vi "ServoControl_myrio_v3_measure.vi"() -> ()   [LabVIEW 2019]
uses:
  <vilib>/Platform/TimedLoop/XDataNode/timing_clust.ctl
  <vilib>/Platform/TimedLoop/XDataNode/nitl_modes.ctl
  <vilib>/Platform/TimedLoop/XDataNode/wakeup.ctl
  <vilib>/Instr/_visa.llb/VISA Configure Serial Port (Instr).vi
  <vilib>/Utility/file.llb/Write Delimited Spreadsheet (DBL).vi
  <vilib>/platform/TimedLoop/XDataNode/XDataNode.xnode
  <vilib>/Platform/TimedLoop/XDataNode/XDNodeRunTimeDep.lvlib
panel:
  in  "Period":dbl
  out "Position Chart":cluster{dbl, dbl}(graph)
  out "Position Graph":cluster{dbl[], dbl[]}[](graph)
  in  "plot freq.":i32=5
  in  "const(f)/sine(t)":bool
  out "iteration":i32
  out "time":dbl
  out "sine position":dbl
  out "read from visa":string
  out "write to visa":string
  in  "const posotion":dbl=180.0
  in  "format (%.3f)":string="%.3f"
  in  "file path (dialog if empty)":path
  in  "Period":i64=5
  in  "stop":bool
  in  "VISA resource name":refnum<visa-resource-name>="ASRL2::INSTR"
  in  "baud rate (9600)":u32=500000
  out "error out":errorcluster
  # "visa setting"
  # "measure time"
  # "status setting"
  # "File save"
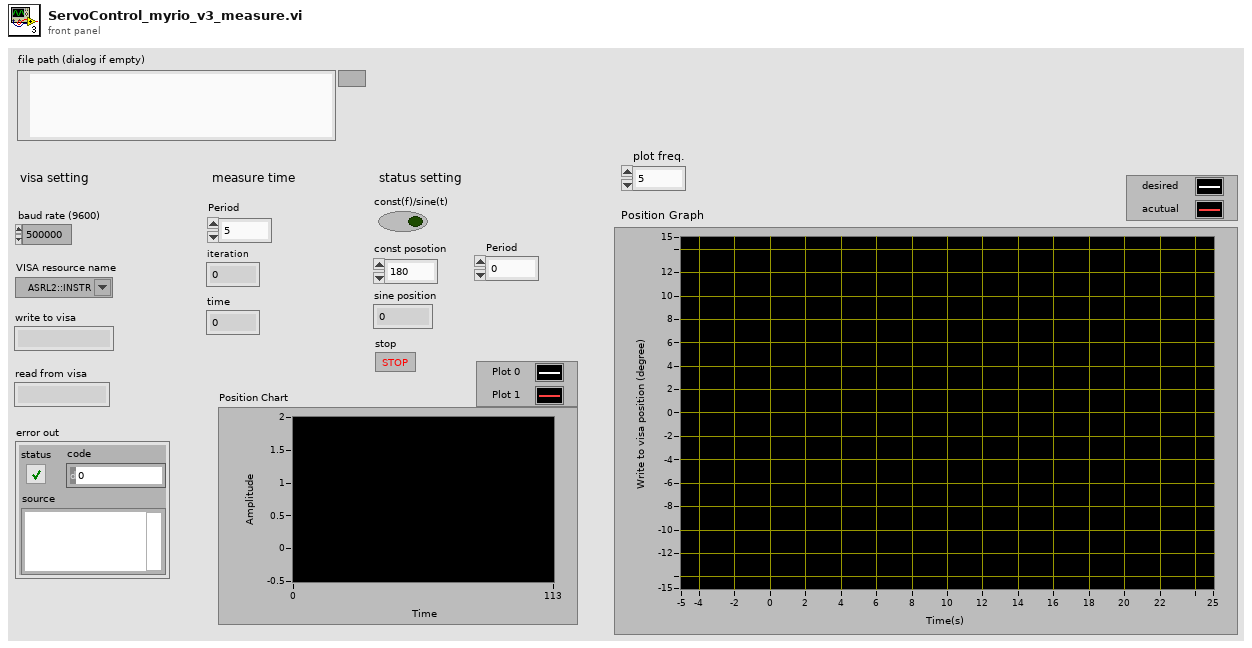
[diagram p1: front panel]
types:
  T1 = typedef "XDNodeRunTimeDep.lvlib/timing_clust.ctl" = cluster{"Expected End [f-1]":u64, "Actual End [f-1]":u64, "Finished Late? [f-1]":bool, "Expected End [i-1]":u64, "Actual End [i-1]":u64, "Finished Late? [i-1]":bool, "Expected Start [i]":u64, "Actual Start [i]":u64, "Expected Start [f]":u64, "Actual Start [f]":u64, "Source Name":string, "Structure Name":string, "Period":i64, "Deadline":i64, "Offset":i64, "Start":i64, "Priority":i32, "Timeout":i32, "Mode":T2, "Wakeup Reason":T3, "Error":errorcluster, "Source Type":string, "Secondary Source Type":string, "Global End Time":u64, "Global Start Time":u64, "Frame Duration":u64, "Iteration Duration":u64, "Assigned CPU":i32, "I/O Scan Engine Mode":u32}
  T2 = typedef "XDNodeRunTimeDep.lvlib/nitl_modes.ctl" = enum32{"No Change", "Process missed periods, maintain original phase", "Discard missed periods, maintain original phase", "Process missed periods, ignore original phase", "Discard missed periods, ignore original phase"}
  T3 = typedef "XDNodeRunTimeDep.lvlib/wakeup.ctl" = enum32{"Normal", "Aborted", "Asynchronous wakeup", "Timing source error", "Timed loop error", "Timeout"}
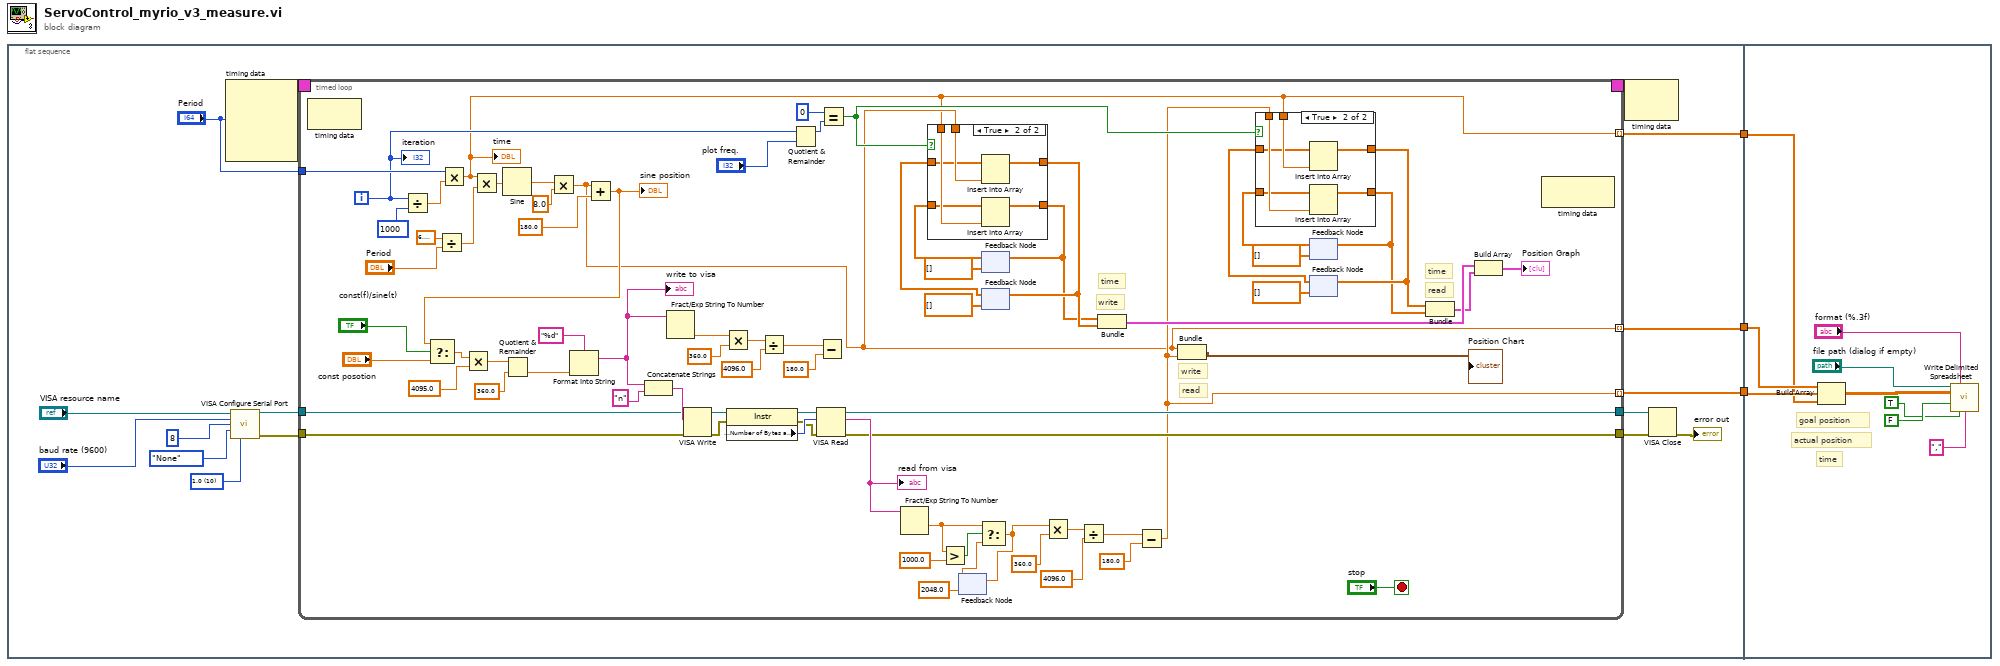
[diagram p0: block diagram]
diagram:
  n1 = flat-sequence {
    tunnel: [w7] -> w3
    tunnel: [w6] -> w2
    tunnel: [w5] -> w1
    tunnel: w3 -> [w118]
    tunnel: w2 -> [w117]
    tunnel: w1 -> [w116]
    frame #0 {
      w14 = u16 10 items=["1.0"=10, "1.5"=15, "2.0"=20] ("stop bits (10: 1 bit)")
      n2 = node-c288("Period") -> (w19:T1)  [unwired: 3 in]
      n3 = call-poly "VISA Configure Serial Port"("VISA resource name"="VISA resource name", "baud rate (9600)"="baud rate (9600)", "data bits (8)"=u16 8, "parity (0:none)"=enum16{"None", "Odd", "Even", "Mark", "Space"}."None", "stop bits (10: 1 bit)"=w14) -> ("VISA resource name out"=w13:refnum<visa-resource-name>, "error out"=w12:errorcluster)  [unwired: 9 in]
      n4 = timed-loop {
        timing: w19 -> [_]
        timing-out: [_] -> w18
        tunnel: "Period" -> [w35]
        tunnel: w12 -> [w36]
        tunnel: [w33] -> w11
        tunnel: w13 -> [w37]
        tunnel: [w32] -> w4
        tunnel: [w30] -> w7 mode=indexing
        tunnel: [w31] -> w6 mode=indexing
        tunnel: [w29] -> w5 mode=indexing
        i -> [w34]
        stop <- "stop" stop-if-true
        # "time"
        # "read"
        # "time"
        # "write"
        # "read"
        # "write"
        n5 = node-c288() -> ()  [unwired: 1 in, 1 out]
        n6 = Divide(x=w34, y=i64 1000) -> (x/y=w70:dbl)
        n7 = Divide(x=6.283185307179586, y="Period") -> (x/y=w20:dbl)
        n8 = Multiply(x=w35, y=w70) -> (x*y=w29:dbl)
        "time" <- w29
        n9 = Multiply(x=w29, y=w20) -> (x*y=w73:dbl)
        n10 = Sine(x=w73) -> (sin(x)=w56:dbl)
        n11 = Multiply(x=w56, y=8.0) -> (x*y=w30:dbl)
        n12 = Add(x=w30, y=180.0) -> (x+y=w68:dbl)
        "sine position" <- w68
        n13 = Select(t=w68, s="const(f)/sine(t)", f="const posotion") -> (s? t:f=w66:dbl)
        n14 = Multiply(x=w66, y=4095.0) -> (x*y=w90:dbl)
        n15 = Quotient & Remainder(x=w90, y=360.0) -> (floor(x/y)=w88:dbl)  [unwired: 1 out]
        n16 = Format Into String(format string="%d", w88) -> (resulting string=w80:string)  [unwired: 2 in, 1 out]
        "write to visa" <- w80
        n17 = Concatenate Strings(w80, "n" ("string")) -> (w92:string)
        n18 = Fract/Exp String To Number(string=w80) -> (number=w79:dbl)  [unwired: 3 in, 1 out]
        n19 = VISA Write(VISA resource name=w37, write buffer=w92, error in (no error)=w36) -> (VISA resource name out=w54:refnum<visa-resource-name>, error out=w53:errorcluster)  [unwired: 1 out]
        n20 = Multiply(x=w79, y=360.0 ("x")) -> (x*y=w77:dbl)
        n21 = property class="Instr"(reference=w54, error in=w53) -> (reference out=w51:refnum<visa-resource-name>, error out=w50:errorcluster, "Serial Settings:Number of Bytes at Serial Port"=w52:u32)
        n22 = Divide(x=w77, y=4096.0) -> (x/y=w83:dbl)
        n23 = Quotient & Remainder(x=w34, y="plot freq.") -> (x-y*floor(x/y)=w61:i32)  [unwired: 1 out]
        n24 = VISA Read(VISA resource name=w51, byte count=w52, error in (no error)=w50) -> (VISA resource name out=w32:refnum<visa-resource-name>, read buffer=w81:string, error out=w33:errorcluster)  [unwired: 1 out]
        "read from visa" <- w81
        n25 = Subtract(x=w83, y=180.0) -> ()  [unwired: 1 out]
        n26 = Equal?(x=0, y=w61) -> (x = y?=w40:bool)
        n27 = Fract/Exp String To Number(string=w81) -> (number=w49:dbl)  [unwired: 3 in, 1 out]
        n28 = Greater?(x=w49, y=1000.0) -> (0:w48:bool)
        n29 = feedback #1(2048.0) -> (w24:dbl)
        n30 = Select(t=w49, s=w48, f=w24) -> (s? t:f=w25:dbl)
        n31 = feedback-in #1(w25) -> ()
        n32 = feedback #2(dbl[] []) -> (w65:dbl[])
        n33 = feedback #3(dbl[] []) -> (w62:dbl[])
        n34 = case shown="True" w40 {
          tunnel: w30 -> [_ w109]
          tunnel: w29 -> [_ w108]
          tunnel: [w103 w107] -> w57
          tunnel: w65 -> [w103 w106]
          tunnel: [w102 w105] -> w58
          tunnel: w62 -> [w102 w104]
          frame False {
          }
          frame True {
            n35 = Insert Into Array(array=w104, new element=w109) -> (w105:dbl[])  [unwired: 1 in]
            n36 = Insert Into Array(array=w106, new element=w108) -> (w107:dbl[])  [unwired: 1 in]
          }
        }
        n37 = feedback-in #2(w57) -> ()
        n38 = feedback-in #3(w58) -> ()
        n39 = Multiply(x=w25, y=360.0 ("x")) -> (x*y=w74:dbl)
        n40 = Divide(x=w74, y=4096.0) -> (x/y=w76:dbl)
        n41 = Bundle(w57, w58) -> (w43:cluster{dbl[], dbl[]})  [unwired: 1 in]
        n42 = Subtract(x=w76, y=180.0) -> (x-y=w31:dbl)
        n43 = Bundle(w30, w31) -> (→"Position Chart":cluster{dbl, dbl})  [unwired: 1 in]
        n44 = feedback #4(dbl[] []) -> (w47:dbl[])
        n45 = feedback #5(dbl[] []) -> (w44:dbl[])
        n46 = case shown="True" w40 {
          tunnel: w29 -> [_ w101]
          tunnel: w31 -> [_ w100]
          tunnel: [w95 w99] -> w38
          tunnel: w47 -> [w95 w98]
          tunnel: [w94 w97] -> w39
          tunnel: w44 -> [w94 w96]
          frame False {
          }
          frame True {
            n47 = Insert Into Array(array=w96, new element=w101) -> (w97:dbl[])  [unwired: 1 in]
            n48 = Insert Into Array(array=w98, new element=w100) -> (w99:dbl[])  [unwired: 1 in]
          }
        }
        n49 = feedback-in #4(w38) -> ()
        n50 = feedback-in #5(w39) -> ()
        n51 = Bundle(w39, w38) -> (w42:cluster{dbl[], dbl[]})  [unwired: 1 in]
        n52 = Build Array(w43, w42) -> (→"Position Graph":cluster{dbl[], dbl[]}[])
        n53 = node-c288() -> ()  [unwired: 1 in, 1 out]
        "iteration" <- w34
      }
      n54 = node-c288(w18) -> ()  [unwired: 1 out]
      n55 = VISA Close(VISA resource name=w4, error in (no error)=w11) -> (error out=→"error out":errorcluster)
    }
    frame #1 {
      # "time"
      # "actual position"
      # "goal position"
      n56 = Build Array(w118, w117, w116) -> (w122:dbl[][])
      n57 = call-poly <vilib>:"Write Delimited Spreadsheet.vi"("file path (dialog if empty)"="file path (dialog if empty)", "format (%.3f)"="format (%.3f)", "2D data"=w122, "append to file? (new file:F)"=FALSE ("transpose? (no:F)"), "transpose? (no:F)"=TRUE ("append to file? (new file:F)"), "delimiter (\\t)"="," ("delimiter (\\t)")) -> ()  [unwired: 8 in, 2 out]
    }
  }
